vi "Host_HoppingScan(XZ_TargetModulation).vi"() -> ()   [LabVIEW 2014]
uses:
  <vilib>/userdefined/High Color/nirio_resource_hc.ctl
  <vilib>/Native 3D Graph/xcontrol/3DPC_SurfacePlot.xctl
  <vilib>/Instr/_visa.llb/VISA Configure Serial Port (Instr).vi
  <vilib>/FPGAPlugInAG/PCIe-7851R/niLvFpga_Open_PCIe-7851R.vi
  <vilib>/rvi/interface/common/dynamic/niFpgaDynamicAddResources.vi
  <vilib>/Utility/error.llb/Error Cluster From Error Code.vi
  <vilib>/rvi/errors/niLvFpgaAdjustHostInterfaceError.vi
  <vilib>/FPGAPlugInAG/Dynamic/niLvFpga_Close_Dynamic.vi
  <vilib>/rvi/interface/nirviOpenFPGA/nirviOpenFPGA.xnode
  FPGA Bitfiles/XZFPGAWithinHopp_FPGATarget_HoppingStep(Nonl_XxebUGwmqxw.lvbitx
  <vilib>/rvi/interface/nirviReadWriteControl/nirviReadWriteControl.xnode
  <vilib>/rvi/interface/nirviMethod/nirviMethod.xnode
  <vilib>/rvi/interface/nirviCloseFPGA/nirviCloseFPGA.xnode
  NiFpgaLv.dll
  <vilib>/rvi/interface/Simulation/niFpgaSimulationCallBeginRW.vi
  <vilib>/FPGAPlugInAG/Dynamic/niLvFpga_ReadFifo_Dynamic.vi
  <vilib>/rvi/errors/niLvFpgaMergeErrorWithErrorCode.vi
  <vilib>/FPGAPlugInAG/Dynamic/niLvFpga_StopFifo_Dynamic.vi
panel:
  in  "LowPassFilter":i32
  out "XGetNum":u32
  in  "BottomSleep us":i32
  in  "UpperSleep us":i32
  out "SecElapsed s":dbl
  in  "UseCompensation":bool
  in  "Compensation / line":i32
  in  "RelativeWithdraw index":i32
  out "YPresPos":i32
  out "XBuffer":u32
  out "Waveform Chart":i16[](graph)
  out "3D Graph":refnum<class "Base Datatype.lvclass">[](xcontrol)
  in  "stop":bool
  in  "ZOffset index":i32
  out "YPos?":dbl
  in  "YNum":i16
  in  "XNum":i16
  in  "YStepLen um":dbl format="%#_13g"
  in  "XStepMultiplier / 0.5nm":i16
  in  "XInitPos um":dbl format="%#_13g"
  in  "YInitPos um":dbl format="%#_13g"
  in  "PIXZ":T1
  out "ERR?":string
  in  "PIYDigital":refnum<visa-resource-name>
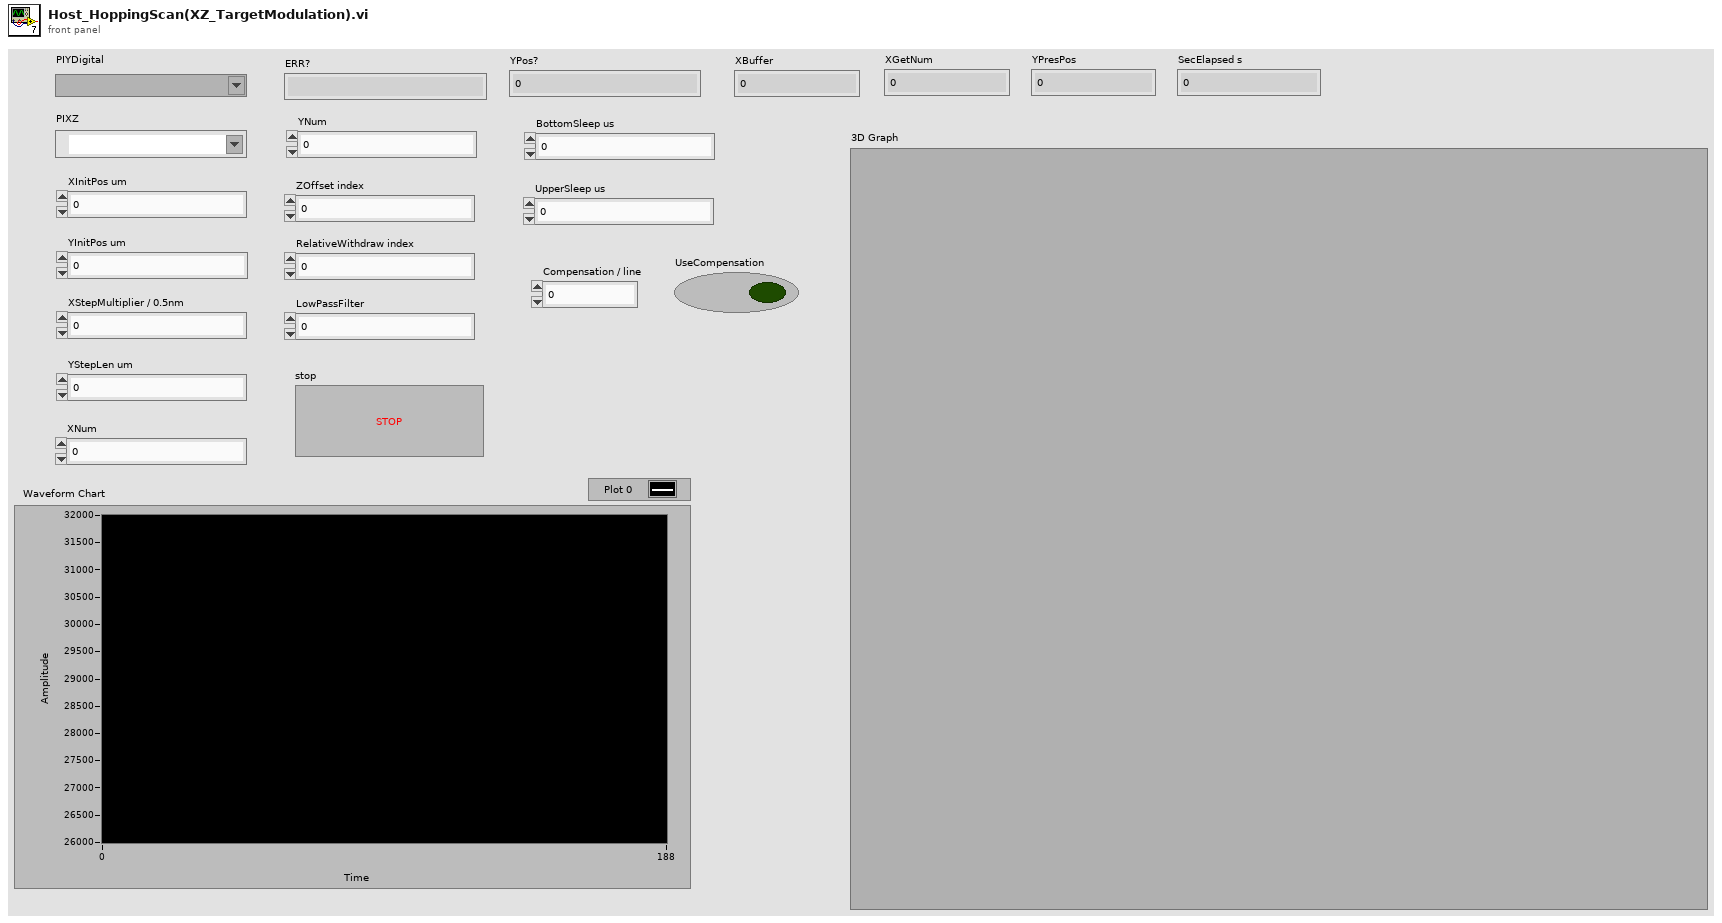
[diagram p1: front panel]
types:
  T1 = typedef "nirio_resource_hc.ctl" = tag
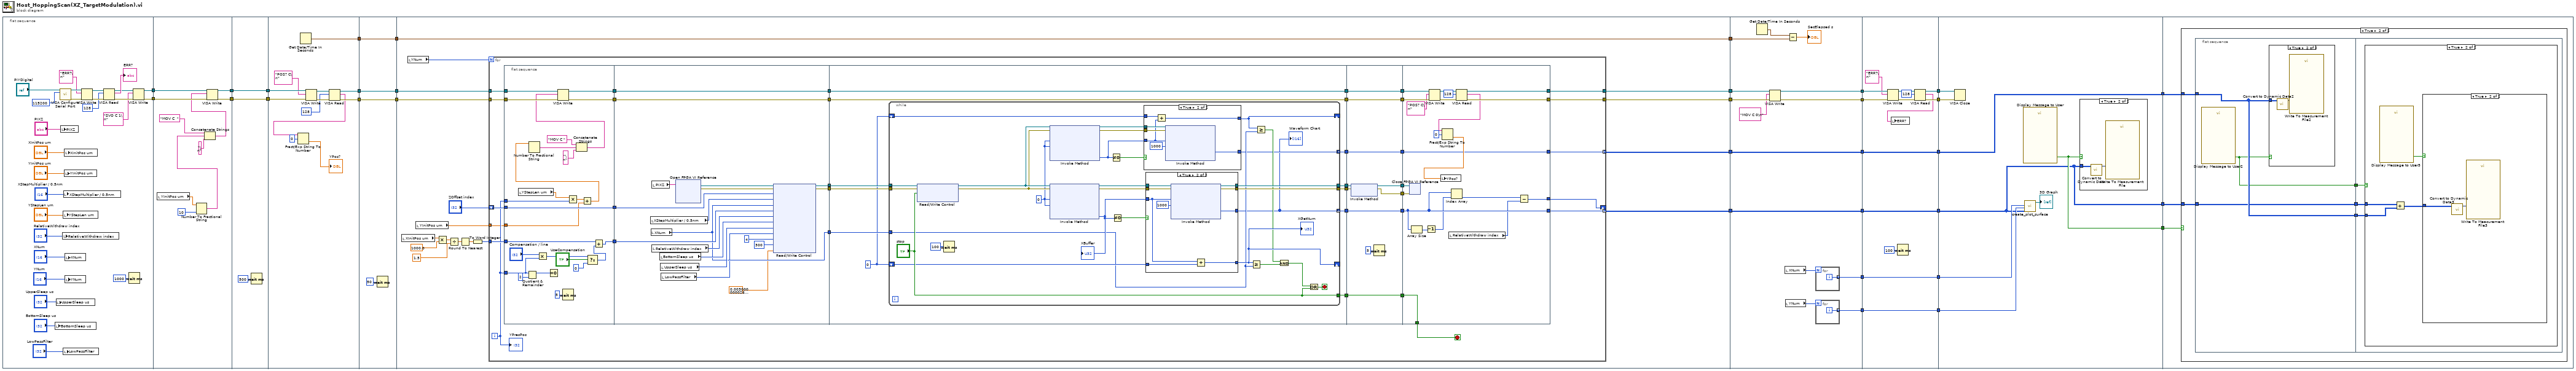
[diagram p0: block diagram]
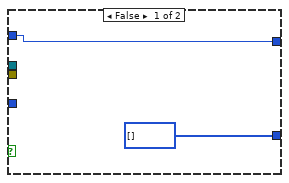
[diagram p2: hidden frame]
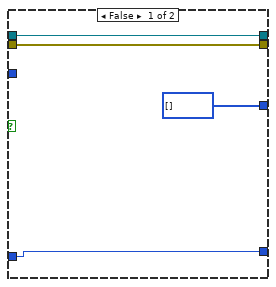
[diagram p3: hidden frame]
diagram:
  n1 = flat-sequence {
    tunnel: [w38] -> w32
    tunnel: [w37] -> w31
    tunnel: w32 -> [w68]
    tunnel: w31 -> [w67]
    tunnel: [w63] -> w30
    tunnel: [w62] -> w29
    tunnel: w30 -> [w70]
    tunnel: w29 -> [w69]
    tunnel: [w70] -> w28
    tunnel: [w69] -> w27
    tunnel: w28 -> [w83]
    tunnel: w27 -> [w82]
    tunnel: [w77] -> w26
    tunnel: [w76] -> w25
    tunnel: [w72] -> w10
    tunnel: w26 -> [w86]
    tunnel: w25 -> [w85]
    tunnel: [w86] -> w24
    tunnel: [w85] -> w23
    tunnel: [w84] -> w11
    tunnel: w10 -> [w84]
    tunnel: w24 -> [w103]
    tunnel: w23 -> [w102]
    tunnel: [w94] -> w22
    tunnel: [w93] -> w21
    tunnel: [w92] -> w16
    tunnel: w11 -> [w89]
    tunnel: [w89] -> w9
    tunnel: [w88] -> w6
    tunnel: w22 -> [w288]
    tunnel: w21 -> [w287]
    tunnel: [w285] -> w20
    tunnel: [w284] -> w19
    tunnel: w16 -> [w281]
    tunnel: [w282] -> w15
    tunnel: [w281] -> w12
    tunnel: w9 -> [w280]
    tunnel: [w277] -> w7
    tunnel: w6 -> [w277]
    tunnel: [w275] -> w2
    tunnel: w20 -> [w304]
    tunnel: w19 -> [w303]
    tunnel: [w298] -> w18
    tunnel: [w297] -> w17
    tunnel: w15 -> [w294]
    tunnel: [w294] -> w14
    tunnel: [w293] -> w13
    tunnel: w12 -> [w293]
    tunnel: [w292] -> w8
    tunnel: w7 -> [w292]
    tunnel: [w291] -> w3
    tunnel: w2 -> [w291]
    tunnel: w18 -> [w312]
    tunnel: w17 -> [w311]
    tunnel: w14 -> [w309]
    tunnel: w13 -> [w305]
    tunnel: w8 -> [w307]
    tunnel: [w308] -> w5
    tunnel: [w307] -> w4
    tunnel: w3 -> [w306]
    tunnel: [w305] -> w1
    tunnel: w5 -> [w315]
    tunnel: w4 -> [w317]
    tunnel: w1 -> [w316]
    frame #0 {
      n2 = local write "BottomSleep us"("BottomSleep us") -> ()
      n3 = local write "UpperSleep us"("UpperSleep us") -> ()
      n4 = call-poly "VISA Configure Serial Port"("VISA resource name"="PIYDigital", "baud rate (9600)"=u32 115200) -> ("VISA resource name out"=w56:refnum<visa-resource-name>, "error out"=w55:errorcluster)  [unwired: 12 in]
      n5 = local write "PIXZ"("PIXZ") -> ()
      n6 = local write "RelativeWithdraw index"("RelativeWithdraw index") -> ()
      n7 = local write "YStepLen um"("YStepLen um") -> ()
      n8 = local write "LowPassFilter"("LowPassFilter") -> ()
      n9 = local write "XStepMultiplier / 0.5nm"("XStepMultiplier / 0.5nm") -> ()
      n10 = local write "YInitPos um"("YInitPos um") -> ()
      n11 = local write "XInitPos um"("XInitPos um") -> ()
      n12 = local write "XNum"("XNum") -> ()
      n13 = local write "YNum"("YNum") -> ()
      n14 = VISA Write(VISA resource name=w56, write buffer="ERR?\n", error in (no error)=w55) -> (VISA resource name out=w53:refnum<visa-resource-name>, error out=w52:errorcluster)  [unwired: 1 out]
      n15 = VISA Read(VISA resource name=w53, byte count=u32 128, error in (no error)=w52) -> (VISA resource name out=w40:refnum<visa-resource-name>, read buffer=→"ERR?":string, error out=w39:errorcluster)  [unwired: 1 out]
      n16 = Wait (ms)(milliseconds to wait=u32 1000) -> ()  [unwired: 1 out]
      n17 = VISA Write(VISA resource name=w40, write buffer="SVO C 1\n", error in (no error)=w39) -> (VISA resource name out=w38:refnum<visa-resource-name>, error out=w37:errorcluster)  [unwired: 1 out]
    }
    frame #1 {
      n18 = local read "YInitPos um"() -> (w61:dbl)
      n19 = Number To Fractional String(number=w61, precision (6)=i16 10) -> (F-format string=w59:string)  [unwired: 2 in]
      n20 = Concatenate Strings("MOV C  " ("write buffer"), w59, "\n" ("string")) -> (w64:string)
      n21 = VISA Write(VISA resource name=w68, write buffer=w64, error in (no error)=w67) -> (VISA resource name out=w63:refnum<visa-resource-name>, error out=w62:errorcluster)  [unwired: 1 out]
    }
    frame #2 {
      n22 = Wait (ms)(milliseconds to wait=u32 500) -> ()  [unwired: 1 out]
    }
    frame #3 {
      n23 = Get Date/Time In Seconds() -> (seconds since 1Jan1904=w72:timestamp)
      n24 = VISA Write(VISA resource name=w83, write buffer="POS? C\n", error in (no error)=w82) -> (VISA resource name out=w80:refnum<visa-resource-name>, error out=w79:errorcluster)  [unwired: 1 out]
      n25 = VISA Read(VISA resource name=w80, byte count=u32 128, error in (no error)=w79) -> (VISA resource name out=w77:refnum<visa-resource-name>, read buffer=w75:string, error out=w76:errorcluster)  [unwired: 1 out]
      n26 = Fract/Exp String To Number(string=w75, offset=0) -> (number=→"YPos?":dbl)  [unwired: 2 in, 1 out]
    }
    frame #4 {
      n27 = Wait (ms)(milliseconds to wait=u32 50) -> ()  [unwired: 1 out]
    }
    frame #5 {
      n28 = local read "XInitPos um"() -> (w96:dbl)
      n29 = local read "YNum"() -> (w104:i16)
      n30 = local read "YInitPos um"() -> (w90:dbl)
      n31 = Multiply(x=w96, y=1000.0) -> (x*y=w98:dbl)
      n32 = Divide(x=w98, y=1.5) -> (x/y=w100:dbl)
      n33 = Round To Nearest(number=w100) -> (nearest integer value=w101:dbl)
      n34 = To Word Integer(number=w101) -> (16bit integer=w95:i16)
      n35 = for {
        N: w104 -> [_]
        tunnel: w103 -> [w139]
        tunnel: w102 -> [w138]
        tunnel: w95 -> [w132]
        tunnel: [w124] -> w94
        tunnel: [w123] -> w93
        tunnel: [w111] -> w92 mode=indexing
        shift-right: [w112] -> _
        shift-left: "ZOffset index" -> [w114]
        tunnel: w90 -> [w108]
        tunnel: [w105] -> w88 mode=indexing
        i -> [w113]
        stop <- w118 stop-if-true
        n36 = flat-sequence {
          tunnel: w139 -> [w163]
          tunnel: w138 -> [w162]
          tunnel: w113 -> [w164]
          tunnel: [w161] -> w137
          tunnel: [w160] -> w136
          tunnel: [w146] -> w133
          tunnel: w132 -> [w147]
          tunnel: [w154] -> w115
          tunnel: w114 -> [w154]
          tunnel: w113 -> [w144]
          tunnel: w108 -> [w149]
          tunnel: [w179] -> w135
          tunnel: [w178] -> w134
          tunnel: [w175] -> w131
          tunnel: [w174] -> w130
          tunnel: [w169] -> w127
          tunnel: w115 -> [w173]
          tunnel: w133 -> [w176]
          tunnel: w136 -> [w178]
          tunnel: w137 -> [w179]
          tunnel: w135 -> [w193]
          tunnel: w134 -> [w192]
          tunnel: w131 -> [w186]
          tunnel: w130 -> [w185]
          tunnel: [w193] -> w129
          tunnel: [w192] -> w128
          tunnel: w127 -> [w191]
          tunnel: [w190] -> w126
          tunnel: [w189] -> w125
          tunnel: [w188] -> w120
          tunnel: [w187] -> w116
          tunnel: [w183] -> w106
          tunnel: w129 -> [w253]
          tunnel: w128 -> [w252]
          tunnel: w126 -> [w248]
          tunnel: w125 -> [w247]
          tunnel: [w253] -> w122
          tunnel: [w252] -> w121
          tunnel: w120 -> [w250]
          tunnel: [w250] -> w119
          tunnel: [w249] -> w117
          tunnel: w116 -> [w249]
          tunnel: [w246] -> w110
          tunnel: [w245] -> w109
          tunnel: [w244] -> w107
          tunnel: w106 -> [w244]
          tunnel: [w271] -> w112
          tunnel: [w273] -> w123
          tunnel: [w274] -> w124
          tunnel: [w270] -> w111
          tunnel: w109 -> [w255]
          tunnel: w110 -> [w256]
          tunnel: w117 -> [w270]
          tunnel: [w261] -> w118
          tunnel: w119 -> [w261]
          tunnel: w121 -> [w268]
          tunnel: w122 -> [w269]
          tunnel: w107 -> [w254]
          tunnel: [w254] -> w105
          frame #0 {
            n37 = local read "YStepLen um"() -> (w159:dbl)
            n38 = Quotient & Remainder(x=w144, y=2) -> (x-y*floor(x/y)=w152:i32)  [unwired: 1 out]
            n39 = Multiply(x="Compensation / line", y=w144) -> (x*y=w143:i32)
            n40 = Equal To 0?(x=w152) -> ()  [unwired: 1 out]
            n41 = Wait (ms)(milliseconds to wait=u32 5) -> ()  [unwired: 1 out]
            n42 = Multiply(x=w159, y=w164) -> (x*y=w150:dbl)
            n43 = Add(x=w150, y=w149) -> (x+y=w148:dbl)
            n44 = Number To Fractional String(number=w148) -> (F-format string=w158:string)  [unwired: 3 in]
            n45 = Concatenate Strings("MOV C " ("string"), w158, "\n" ("string")) -> (w155:string)
            n46 = VISA Write(VISA resource name=w163, write buffer=w155, error in (no error)=w162) -> (VISA resource name out=w161:refnum<visa-resource-name>, error out=w160:errorcluster)  [unwired: 1 out]
            n47 = Select(t=w143, s="UseCompensation", f=0) -> (s? t:f=w140:i32)
            n48 = Add(x=w147, y=w140) -> (x+y=w146:i32)
          }
          frame #1 {
            n49 = local read "XStepMultiplier / 0.5nm"() -> (w177:i16)
            n50 = local read "XNum"() -> (w169:i16)
            n51 = local read "PIXZ"() -> (w182:T1)
            n52 = local read "RelativeWithdraw index"() -> (w172:i32)
            n53 = local read "BottomSleep us"() -> (w171:i32)
            n54 = local read "UpperSleep us"() -> (w170:i32)
            n55 = local read "LowPassFilter"() -> (w168:i32)
            n56 = xnode "Open FPGA VI Reference"("resource name"=w182) -> ("FPGA VI Reference Out"=w181:refnum<k20>, "error out"=w180:errorcluster)  [unwired: 1 in]
            n57 = xnode "Read/Write Control"("FPGA VI Reference In"=w181, "error in"=w180, "ZOffset"=w173, "XStepIndex"=w177, "XNum"=w169, "XOffset"=w176, "RelativeWithdraw"=w172, "BottomSleep us"=w171, "UpperSleep us"=w170, "LowPassFilter"=w168, "ExtraStepIn"=u32 4, "TimeConstant"=u32 300, "threshold"=sgl 0.003) -> ("FPGA VI Reference Out"=w175:refnum<k20>, "error out"=w174:errorcluster)
          }
          frame #2 {
            w184 = 0
            n58 = while {
              tunnel: w186 -> [w215]
              tunnel: w185 -> [w214]
              tunnel: w191 -> [w198]
              tunnel: [w218] -> w190
              tunnel: [w217] -> w189
              tunnel: ["stop"] -> w188
              tunnel: [w194] -> w187 mode=concatenating
              shift-right: [w210] -> _
              shift-left: w184 -> [w211]
              shift-right: [w199] -> _
              shift-left: w184 -> [w201]
              tunnel: [w195] -> w183 mode=concatenating
              stop <- w216 stop-if-true
              w207 = u32 0 ("Number of Elements")
              n59 = xnode "Read/Write Control"("FPGA VI Reference In"=w215, "error in"=w214, "stop"="stop") -> ("FPGA VI Reference Out"=w209:refnum<k20>, "error out"=w208:errorcluster)  [unwired: 1 out]
              n60 = Wait (ms)(milliseconds to wait=u32 100) -> ()  [unwired: 1 out]
              n61 = xnode "Invoke Method"("FPGA VI Reference In"=w209, "error in"=w208, "Number of Elements"=w207, "Timeout (ms)"=w207) -> ("FPGA VI Reference Out"=w220:refnum<k20>, "error out"=w219:errorcluster, "Elements Remaining"=w212:u32)  [unwired: 1 out]
              "XBuffer" <- w212
              n62 = xnode "Invoke Method"("FPGA VI Reference In"=w209, "error in"=w208, "Number of Elements"=w207, "Timeout (ms)"=w207) -> ("FPGA VI Reference Out"=w204:refnum<k20>, "error out"=w203:errorcluster, "Elements Remaining"=w202:u32)  [unwired: 1 out]
              n63 = Not Equal To 0?(x=w202) -> (x != 0?=w205:bool)
              n64 = Not Equal To 0?(x=w212) -> (x != 0?=w206:bool)
              n65 = case shown="True" w205 {
                tunnel: w204 -> [_ w230]
                tunnel: w203 -> [_ w229]
                tunnel: w202 -> [_ w226]
                tunnel: w201 -> [w223 w227]
                tunnel: [w223 w225] -> w199
                tunnel: [i16[] [] ("Data") w224] -> w195
                frame False {
                }
                frame True {
                  n66 = Add(x=w227, y=w226) -> (x+y=w225:u32)
                  n67 = xnode "Invoke Method"("FPGA VI Reference In"=w230, "error in"=w229, "Number of Elements"=w226, "Timeout (ms)"=1000) -> ("Data"=w224:i16[])  [unwired: 3 out]
                }
              }
              n68 = case shown="True" w206 {
                tunnel: w220 -> [w234 w243]
                tunnel: w219 -> [w233 w242]
                tunnel: [w234 w240] -> w218
                tunnel: [w233 w239] -> w217
                tunnel: [i16[] [] ("Data") w238] -> w194
                tunnel: w212 -> [_ w236]
                tunnel: w211 -> [w231 w237]
                tunnel: [w231 w235] -> w210
                frame False {
                }
                frame True {
                  n69 = xnode "Invoke Method"("FPGA VI Reference In"=w243, "error in"=w242, "Number of Elements"=w236, "Timeout (ms)"=1000) -> ("FPGA VI Reference Out"=w240:refnum<k20>, "error out"=w239:errorcluster, "Data"=w238:i16[])  [unwired: 1 out]
                  n70 = Add(x=w236, y=w237) -> (x+y=w235:u32)
                }
              }
              "XGetNum" <- w210
              "Waveform Chart" <- w194
              n71 = Greater Or Equal?(x=w210, y=w198) -> (x >= y?=w200:bool)
              n72 = Greater Or Equal?(x=w199, y=w198) -> (x >= y?=w197:bool)
              n73 = And(x=w197, y=w200) -> (x .and. y?=w196:bool)
              n74 = Or(x=w196, y="stop") -> (x .or. y?=w216:bool)
            }
          }
          frame #3 {
            n75 = xnode "Invoke Method"("FPGA VI Reference In"=w248, "error in"=w247) -> ("FPGA VI Reference Out"=w246:refnum<k20>, "error out"=w245:errorcluster)
            n76 = Wait (ms)(milliseconds to wait=u32 5) -> ()  [unwired: 1 out]
          }
          frame #4 {
            n77 = xnode "Close FPGA VI Reference"("FPGA VI Reference In"=w256, "error in"=w255) -> ()  [unwired: 1 out]
            n78 = Array Size(array=w270) -> (size(s)=w260:i32)
            n79 = Decrement(x=w260) -> (x-1=w259:i32)
            n80 = VISA Write(VISA resource name=w269, write buffer="POS? C\n", error in (no error)=w268) -> (VISA resource name out=w267:refnum<visa-resource-name>, error out=w266:errorcluster)  [unwired: 1 out]
            n81 = local read "RelativeWithdraw index"() -> (w257:i32)
            n82 = Index Array(array=w270, index=w259) -> (element=w258:i16)
            n83 = VISA Read(VISA resource name=w267, byte count=u32 128, error in (no error)=w266) -> (VISA resource name out=w274:refnum<visa-resource-name>, read buffer=w263:string, error out=w273:errorcluster)  [unwired: 1 out]
            n84 = Fract/Exp String To Number(string=w263, offset=0) -> (number=w272:dbl)  [unwired: 2 in, 1 out]
            n85 = local write "YPos?"(w272) -> ()
            n86 = Subtract(x=w258, y=w257) -> (x-y=w271:i32)
          }
        }
        "YPresPos" <- w113
      }
    }
    frame #6 {
      n87 = Get Date/Time In Seconds() -> (seconds since 1Jan1904=w279:timestamp)
      n88 = VISA Write(VISA resource name=w288, write buffer="MOV C 0\n", error in (no error)=w287) -> (VISA resource name out=w285:refnum<visa-resource-name>, error out=w284:errorcluster)  [unwired: 1 out]
      n89 = local read "XNum"() -> (w283:i16)
      n90 = local read "YNum"() -> (w276:i16)
      n91 = Subtract(x=w279, y=w280) -> (x-y=→"SecElapsed s":dbl)
      n92 = for {
        N: w283 -> [_]
        tunnel: [w290] -> w282 mode=indexing
        i -> [w290]
      }
      n93 = for {
        N: w276 -> [_]
        tunnel: [w289] -> w275 mode=indexing
        i -> [w289]
      }
    }
    frame #7 {
      n94 = VISA Write(VISA resource name=w304, write buffer="ERR?\n", error in (no error)=w303) -> (VISA resource name out=w301:refnum<visa-resource-name>, error out=w300:errorcluster)  [unwired: 1 out]
      n95 = Wait (ms)(milliseconds to wait=u32 100) -> ()  [unwired: 1 out]
      n96 = VISA Read(VISA resource name=w301, byte count=u32 128, error in (no error)=w300) -> (VISA resource name out=w298:refnum<visa-resource-name>, read buffer=w296:string, error out=w297:errorcluster)  [unwired: 1 out]
      n97 = local write "ERR?"(w296) -> ()
    }
    frame #8 {
      n98 = VISA Close(VISA resource name=w312, error in (no error)=w311) -> ()  [unwired: 1 out]
      n99 = call "Display Message to User"() -> ("OK"=w308:bool)  [unwired: 10 in, 1 out]
      n100 = call <vilib>:"create_plot_surface.vi"("z matrix"=w305, "y vector"=w306, "x vector"=w309) -> ("plots out"=→"3D Graph":refnum<class "Base Datatype.lvclass">[])  [unwired: 2 in, 6 out]
      n101 = case shown="True" w308 {
        tunnel: w305 -> [_ w314]
        frame False {
        }
        frame True {
          n102 = call "Convert to Dynamic Data"("2D Array"=w314) -> ("Dynamic Data Type"=w313:dynamicdata)  [unwired: 3 in]
          n103 = call "Write To Measurement File"("Signals"=w313) -> ()  [unwired: 16 in, 3 out]
        }
      }
    }
    frame #9 {
      n104 = case shown="True" w315 {
        tunnel: w317 -> [_ w322]
        tunnel: w316 -> [_ w320]
        frame False {
        }
        frame True {
          n105 = flat-sequence {
            tunnel: w322 -> [w325]
            tunnel: [w323] -> w321
            tunnel: w320 -> [w324]
            tunnel: [w325] -> w319
            tunnel: [w324] -> w318
            tunnel: w321 -> [w330]
            tunnel: w319 -> [w329]
            tunnel: w318 -> [w328]
            frame #0 {
              n106 = call "Display Message to User2"() -> ("OK"=w323:bool)  [unwired: 10 in, 1 out]
              n107 = case shown="True" w323 {
                tunnel: w325 -> [_ w327]
                frame False {
                }
                frame True {
                  n108 = call "Convert to Dynamic Data2"("2D Array"=w327) -> ("Dynamic Data Type"=w326:dynamicdata)  [unwired: 3 in]
                  n109 = call "Write To Measurement File2"("Signals"=w326) -> ()  [unwired: 16 in, 3 out]
                }
              }
            }
            frame #1 {
              n110 = case shown="True" w330 {
                tunnel: w329 -> [_ w332]
                tunnel: w328 -> [_ w333]
                frame False {
                }
                frame True {
                  n111 = call "Display Message to User3"() -> ("OK"=w334:bool)  [unwired: 10 in, 1 out]
                  n112 = Add(x=w333, y=w332) -> (x+y=w331:i16[][])
                  n113 = case shown="True" w334 {
                    tunnel: w331 -> [_ w336]
                    frame False {
                    }
                    frame True {
                      n114 = call "Convert to Dynamic Data3"("2D Array"=w336) -> ("Dynamic Data Type"=w335:dynamicdata)  [unwired: 3 in]
                      n115 = call "Write To Measurement File3"("Signals"=w335) -> ()  [unwired: 16 in, 3 out]
                    }
                  }
                }
              }
            }
          }
        }
      }
    }
  }
